vi "Init images and strings.vi"(7 "Type of label":u16(ring) items=["Combo", "String"], 8 "error in (no error)":errorcluster, 9 "String array":refnum<vi>[](array[refnum]), 10 "Image ref array":refnum<vi>[](array[refnum]), 11 "Label array":refnum<vi>[](array[refnum])) -> (0 "error in (no error) 2":errorcluster)   [LabVIEW 2015, in "ZenGage v3.0 UI.lvclass"]
uses:
  ZenGage v3.0 UI.lvclass
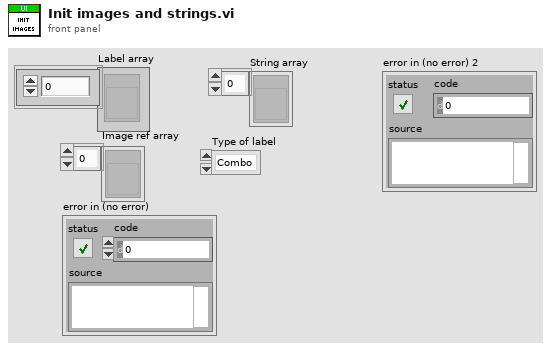
[diagram p1: front panel]
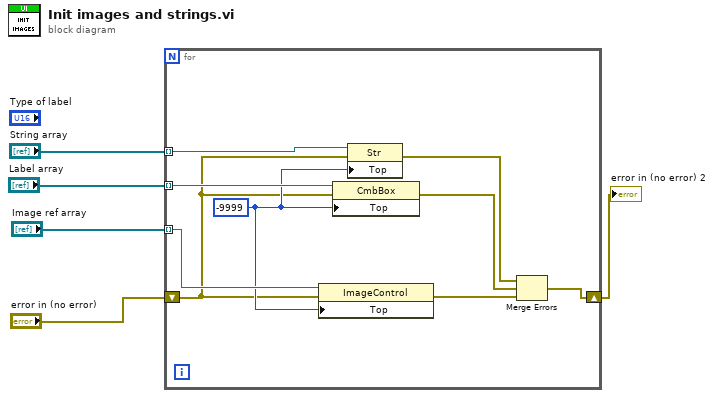
[diagram p0: block diagram]
diagram:
  n1 = for {
    tunnel: "Label array" -> [w14] mode=indexing
    tunnel: "Image ref array" -> [w13] mode=indexing
    shift-right: [w10] -> w2
    shift-left: "error in (no error)" -> [w7]
    tunnel: "String array" -> [w9] mode=indexing
    w8 = -9999 ("Position:Top")
    n2 = property class="ImageControl"(reference=w13, error in=w7, "Top"=w8) -> (error out=w12:errorcluster)  [unwired: 1 out]
    n3 = property class="CmbBox"(reference=w14, error in=w7, "Top"=w8) -> (error out=w11:errorcluster)  [unwired: 1 out]
    n4 = property class="Str"(reference=w9, error in=w7, "Top"=w8) -> (error out=w6:errorcluster)  [unwired: 1 out]
    n5 = Merge Errors(w6, w11, w12) -> (w10:errorcluster)
  }
  "error in (no error) 2" <- w2
